vi "GetVoltage.vi"(4 "error in":errorcluster, 5 "connection ID":refnum<k5>) -> (0 "Voltage":string, 1 "error out":errorcluster, 2 "connection ID out":refnum<k5>, 3 "Answer":bool)   [LabVIEW 2013]
panel:
  out "читаю hex":string
  out "читаю текст":string
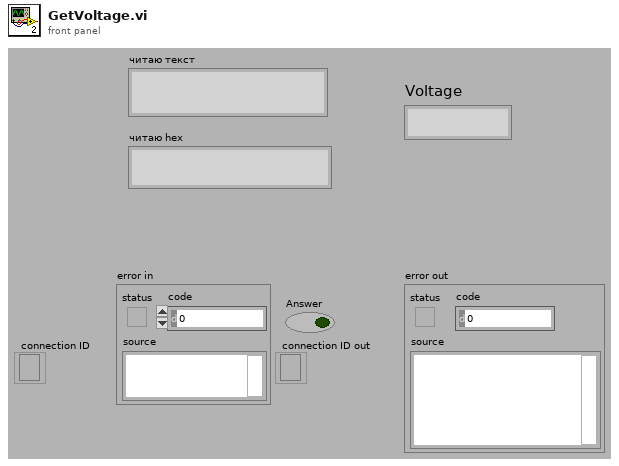
[diagram p1: front panel]
types:
  T1 = enum16{"Standard", "Buffered", "CRLF", "Immediate"}
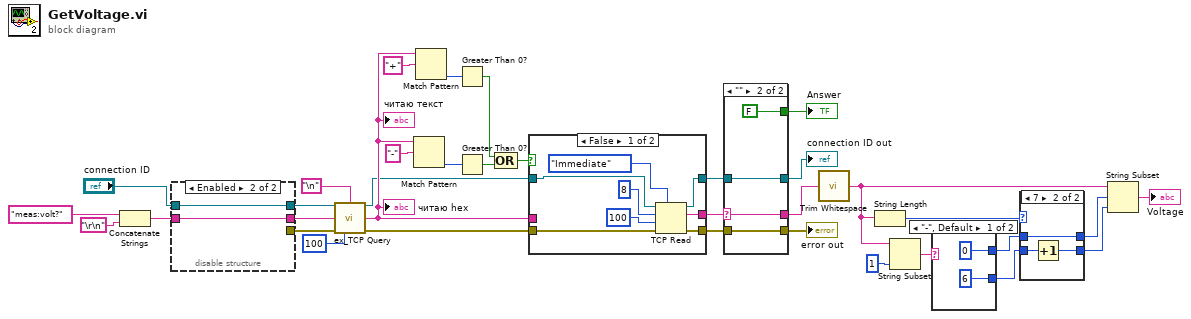
[diagram p0: block diagram]
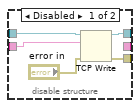
[diagram p2: hidden frame]
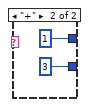
[diagram p4: hidden frame]
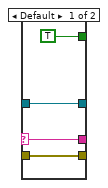
[diagram p6: hidden frame]
diagram:
  n1 = Concatenate Strings("meas:volt?" ("data in"), "\r\n") -> (w33:string)
  n2 = disable-structure shown="Enabled" {
    disable-tunnel: "connection ID" -> [w39 w41]
    disable-tunnel: w33 -> [w38 w42]
    disable-tunnel: [w37 _] -> w8
    disable-tunnel: [w36 w41] -> w7
    disable-tunnel: [_ w42] -> w6
    frame Disabled {
      n3 = TCP Write(connection ID=w39, data in=w38, error in (no error)="error in") -> (connection ID out=w36:refnum<k5>, error out=w37:errorcluster)  [unwired: 2 out]
    }
    frame Enabled {
    }
  }
  n4 = call "ex_TCP Query.vi"("TCP Network Connection in"=w7, "Termination character"="\n", "Query string"=w6, "error in (no error)"=w8, "Initial byte timeout ms (1000)"=100) -> ("TCP Network Connection out"=w3:refnum<k5>, "Message data out"=w4:string, "error out"=w5:errorcluster)  [unwired: 7 in, 1 out]
  "читаю hex" <- w4
  "читаю текст" <- w4
  n5 = Match Pattern(string=w4, regular expression="-") -> (offset past match=w22:i32)  [unwired: 1 in, 3 out]
  n6 = Match Pattern(string=w4, regular expression="+") -> (offset past match=w30:i32)  [unwired: 1 in, 3 out]
  n7 = Greater Than 0?(x=w30) -> (x > 0?=w21:bool)
  n8 = Greater Than 0?(x=w22) -> (x > 0?=w20:bool)
  n9 = Compound Arithmetic op=OR(w21, w20) -> (w19:bool)
  n10 = case shown="False" w19 {
    tunnel: w4 -> [_ w53]
    tunnel: [w47 w53] -> w26
    tunnel: [w45 w51] -> w25
    tunnel: w5 -> [w46 w51]
    tunnel: w3 -> [w48 w52]
    tunnel: [w43 w52] -> w24
    frame False {
      n11 = TCP Read(connection ID=w48, bytes to read=8, error in (no error)=w46, 7:T1."Immediate" ("mode (standard)"), 9:100 ("timeout ms (25000)")) -> (connection ID out=w43:refnum<k5>, data out=w47:string, error out=w45:errorcluster)
    }
    frame True {
    }
  }
  n12 = case shown="\"\"" w26 {
    selector: w26 -> [w57 w61]
    tunnel: [w57 w61] -> w9
    tunnel: [TRUE FALSE] -> w27
    tunnel: w25 -> [w55 w59]
    tunnel: [w55 w59] -> w28
    tunnel: w24 -> [w54 w58]
    tunnel: [w54 w58] -> w29
    frame Default {
    }
    frame "" {
    }
  }
  "Answer" <- w27
  "connection ID out" <- w29
  "error out" <- w28
  n13 = call <vilib>:"Trim Whitespace.vi"("string"=w9) -> ("trimmed string"=w16:string)  [unwired: 1 in]
  n14 = String Length(string=w16) -> (length=w15:i32)
  n15 = String Subset(string=w16, length (rest)=1 ("length (rest)")) -> (substring=w18:string)  [unwired: 1 in]
  n16 = case shown="\"-\", Default" w18 {
    tunnel: [0 ("length (rest)") 1 ("length (rest)")] -> w12
    tunnel: [6 ("length (rest)") 3 ("length (rest)")] -> w14
    frame "-", Default {
    }
    frame "+" {
    }
  }
  n17 = case shown="7" w15 {
    tunnel: w14 -> [w67 w70]
    tunnel: [w67 w69] -> w13
    tunnel: w12 -> [w66 w68]
    tunnel: [w66 w68] -> w11
    frame 6, Default {
    }
    frame 7 {
      n18 = Increment(x=w70) -> (x+1=w69:i32)
    }
  }
  n19 = String Subset(string=w16, offset (0)=w11, length (rest)=w13) -> (substring=→"Voltage":string)
